vi "test2-MacroWithSubMessages.vi"(8 "error in":errorcluster, 11 "TestCase in":refnum<class "testcase-CSMResponse.lvclass">) -> (0 "error out":errorcluster, 3 "TestCase out":refnum<class "testcase-CSMResponse.lvclass">)   [LabVIEW 2017, in "testcase-CSMResponse.lvclass"]
uses:
  testcase-CSMResponse.lvclass
  0c6454a9-3719-4e31-9ff6-45b39d38beb6.vi
  <vilib>/addons/_JKI Toolkits/VI Tester/TestCase.llb/TestCase.lvclass
  src/user.lib/_NEVSTOP/Communicable State Machine(CSM)/Communicable State Machine.lvlib
  CSM/CSM-Testcase.lvlib
  C:/Program Files (x86)/National Instruments/LabVIEW 2017/vi.lib/addons/_JKI Toolkits/VI Tester/TestCase.llb/TestCase.lvclass
panel:
  out "Loopcount":i32
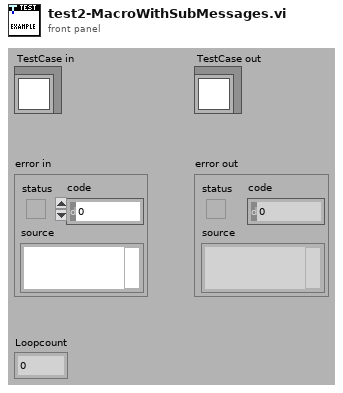
[diagram p1: front panel]
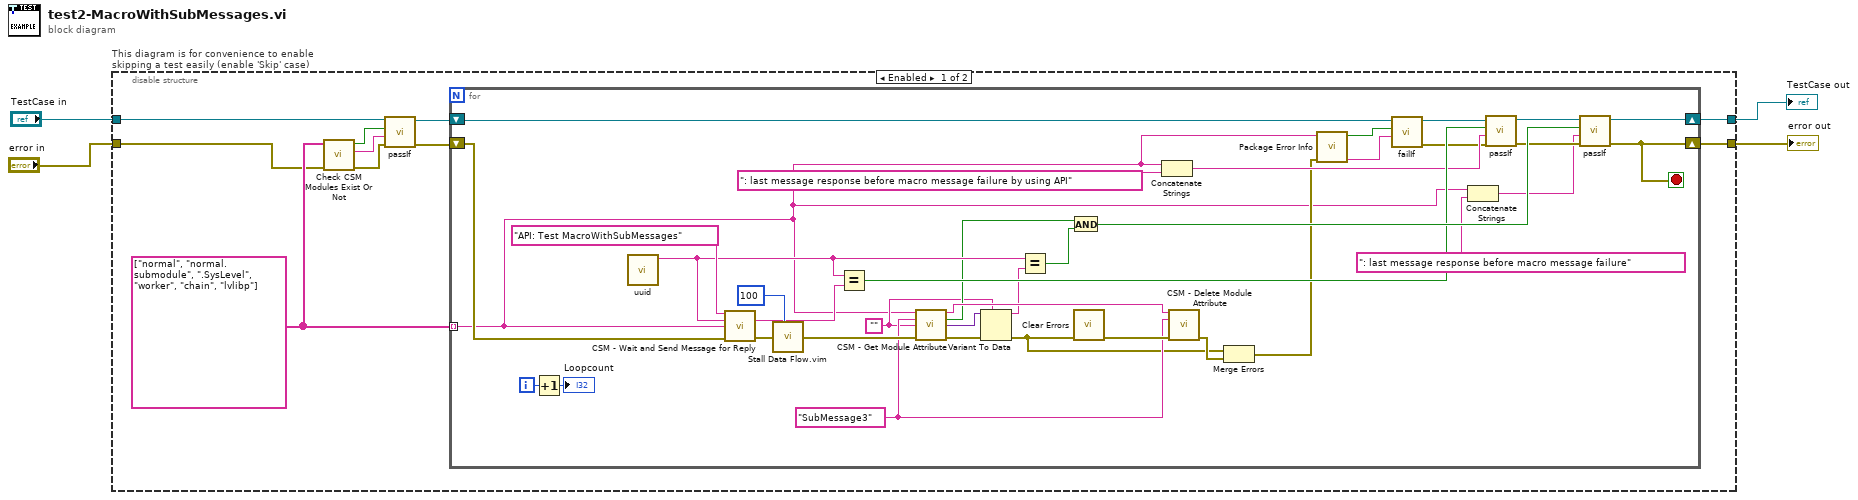
[diagram p0: block diagram]
diagram:
  n1 = disable-structure "This diagram is for convenience to enable skipping a test easily (enable 'Skip' case)" shown="Enabled" {
    disable-tunnel: "TestCase in" -> [w8 w55]
    disable-tunnel: [w14 w53] -> w1
    disable-tunnel: [w13 w54] -> w3
    disable-tunnel: "error in" -> [w6 w52]
    frame Enabled {
      w9 = string[] ["normal", "normal.submodule", ".SysLevel", "worker", "chain", "lvlibp"]
      n2 = call "Check CSM Modules Exist Or Not.vi"("error in"=w6, "CSM names in"=w9) -> ("error out"=w10:errorcluster, "Debug string"=w11:string, "All Modules Exist?"=w12:bool)  [unwired: 7 in]
      n3 = call-dynamic "passIf.vi"("error in (no error)"=w10, "message (\"\")"=w11, "pass"=w12, "TestCase in"=w8) -> ("error out"=w5:errorcluster, "TestCase out"=w7:refnum<class "testcase-CSMResponse.lvclass">)  [unwired: 6 in]
      n4 = for {
        tunnel: w9 -> [w15] mode=indexing
        shift-right: [w43] -> w14
        shift-left: w7 -> [w19]
        shift-right: [w42] -> w13
        shift-left: w5 -> [w36]
        i -> [w51]
        stop <- w42 stop-if-true
        w29 = ""
        w34 = "SubMessage3" ("Attribute")
        n5 = Increment(x=w51) -> (x+1=→"Loopcount":i32)
        n6 = call "uuid.vi"() -> ("UUID"=w40:string)  [unwired: 11 in]
        n7 = call "CSM - Wait and Send Message for Reply.vi"("State"="API: Test MacroWithSubMessages", "Arguments (\"\")"=w40, "Target Module"=w15, "Error In (No Error)"=w36) -> ("Response"=w41:string, "error out"=w49:errorcluster)  [unwired: 8 in, 2 out]
        n8 = call "Stall Data Flow.vim"("value in"=w49, "milliseconds to wait"=u32 100) -> ("value out"=w35:errorcluster)  [unwired: 1 out]
        n9 = Equal?(x=w40, y=w41) -> (x = y?=w39:bool)
        n10 = call "CSM - Get Module Attribute.vi"("CSM Name"=w15, "Attribute"=w34, "Default Value (Empty Variant)"=w29, "Error In"=w35) -> ("CSM Name (Dup)"=w33:string, "Found"=w32:bool, "Value"=w30:variant, "error out"=w31:errorcluster)  [unwired: 7 in, 1 out]
        n11 = Variant To Data(error in=w31, type=w29, Variant=w30) -> (data=w28:string, error out=w26:errorcluster)
        n12 = Equal?(x=w40, y=w28) -> (x = y?=w46:bool)
        n13 = And(x=w32, y=w46) -> (x .and. y?=w45:bool)
        n14 = call <vilib>:"Clear Errors.vi"("error in (no error)"=w26) -> ("error out"=w44:errorcluster)  [unwired: 5 in, 1 out]
        n15 = Concatenate Strings(w15, ": last message response before macro message failure by using API" ("string")) -> (w24:string)
        n16 = call "CSM - Delete Module Attribute.vi"("CSM Name"=w33, "Attribute"=w34, "Error In"=w44) -> ("error out"=w27:errorcluster)  [unwired: 9 in, 3 out]
        n17 = Merge Errors(w26, w27) -> (w16:errorcluster)
        n18 = call "Package Error Info.vi"("error in"=w16, "String in"=w15) -> ("packed error info out"=w20:string, "error status"=w21:bool)  [unwired: 8 in]
        n19 = call-dynamic "failIf.vi"("message (\"\")"=w20, "fail"=w21, "TestCase in"=w19) -> ("error out"=w17:errorcluster, "TestCase out"=w18:refnum<class "testcase-CSMResponse.lvclass">)  [unwired: 7 in]
        n20 = Concatenate Strings(w15, ": last message response before macro message failure" ("string")) -> (w22:string)
        n21 = call-dynamic "passIf.vi"("error in (no error)"=w17, "message (\"\")"=w24, "pass"=w39, "TestCase in"=w18) -> ("error out"=w37:errorcluster, "TestCase out"=w38:refnum<class "testcase-CSMResponse.lvclass">)  [unwired: 6 in]
        n22 = call-dynamic "passIf.vi"("error in (no error)"=w37, "message (\"\")"=w22, "pass"=w45, "TestCase in"=w38) -> ("error out"=w42:errorcluster, "TestCase out"=w43:refnum<class "testcase-CSMResponse.lvclass">)  [unwired: 6 in]
      }
    }
    frame Disabled {
      # "skip test result while test is under development"
      n23 = call <vilib>:"skip.vi"("error in (no error)"=w52, "TestCase in"=w55) -> ("error out"=w54:errorcluster, "TestCase out"=w53:refnum<class "testcase-CSMResponse.lvclass">)  [unwired: 8 in]
    }
  }
  "error out" <- w3
  "TestCase out" <- w1
